vi "Angle_RT_test.vi"() -> ()   [LabVIEW 2021]
uses:
  <vilib>/DAQmx/read.llb/DAQmx Read (Digital 2D U32 NChan NSamp).vi
  <vilib>/Analysis/baseanly.llb/Mean (DBL).vi
  <vilib>/DAQmx/miscellaneous.llb/DAQmx Fill In Error Info.vi
  <vilib>/Analysis/NI_AALBase.lvlib
panel:
  out "Numeric":i32
  in  "stop":bool
  out "error out":errorcluster
  in  "Zero Angle":dbl[](array[numeric])=[-16.79, 2.64, -15.0, 3.7]
  out "Encoder Raw Outputs":dbl[][](array[numeric])
  out "Encoder Mean Outputs":dbl[](array[numeric])
  in  "Input Rate (Hz)":dbl
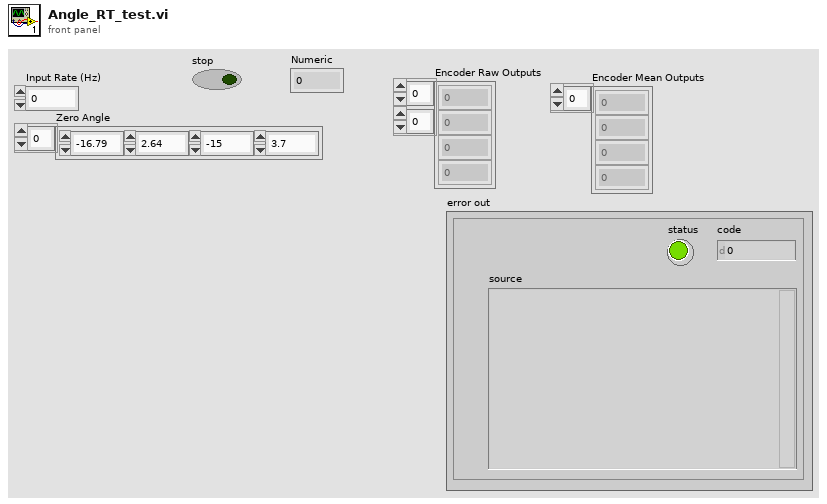
[diagram p1: front panel]
types:
  T1 = cluster{"Csn task out":refnum<k21>, "CLK task out":refnum<k21>, "D0 task out":refnum<k21>}
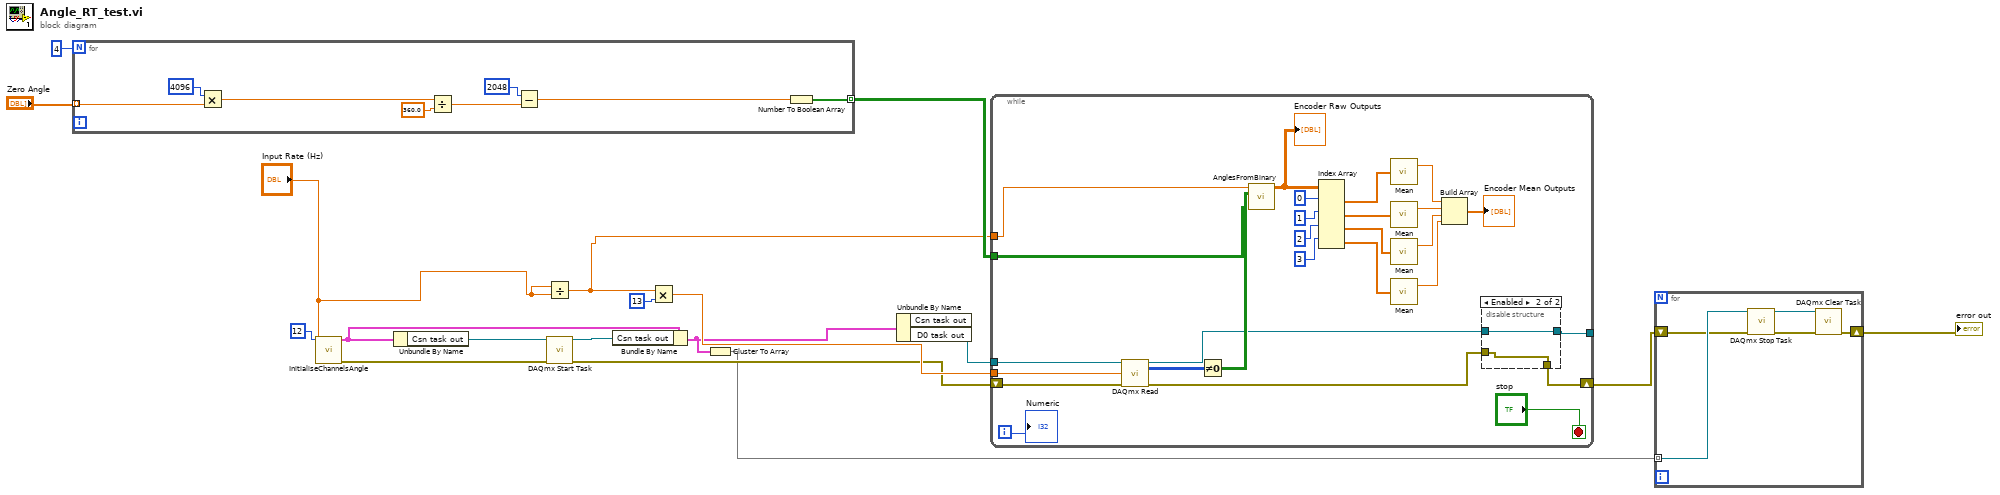
[diagram p0: block diagram]
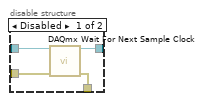
[diagram p2: hidden frame]
diagram:
  n1 = for {
    N: 4 -> [_]
    tunnel: [w22] -> w9 mode=indexing
    tunnel: "Zero Angle" -> [w25] mode=indexing
    n2 = Multiply(x=4096, y=w25) -> (x*y=w26:dbl)
    n3 = Divide(x=w26, y=360.0) -> (x/y=w20:dbl)
    n4 = Subtract(x=2048, y=w20) -> (x-y=w19:dbl)
    n5 = Number To Boolean Array(number=w19) -> (Boolean array=w22:bool[])
  }
  n6 = call "InitialiseChannelsAngle.vi"("Number of data bits"=12, "Fs"="Input Rate (Hz)") -> ("output cluster"=w13:T1, "error out"=w14:errorcluster)  [unwired: 12 in]
  n7 = Unbundle By Name(w13) -> ("Csn task out"=w18:refnum<k21>)
  n8 = Divide(x="Input Rate (Hz)", y="Input Rate (Hz)") -> (x/y=w8:dbl)
  n9 = call <vilib>:"DAQmx Start Task.vi"("task/channels in"=w18, "error in"=w14) -> ("task out"=w17:refnum<k21>, "error out"=w6:errorcluster)  [unwired: 12 in]
  n10 = Bundle By Name(cluster=w13, "Csn task out"=w17) -> (w2:T1)
  n11 = Multiply(x=w8, y=13) -> (x*y=w7:dbl)
  n12 = Cluster To Array(cluster=w2) -> (array=w4:refnum<k21>[])
  n13 = Unbundle By Name(w2) -> ("D0 task out"=w1:refnum<k21>)  [unwired: 1 out]
  n14 = while {
    tunnel: w9 -> [w37]
    tunnel: w8 -> [w36]
    tunnel: w7 -> [w35]
    tunnel: w1 -> [w30]
    shift-right: [w31] -> w5
    shift-left: w6 -> [w34]
    tunnel: [w27] -> _
    i -> [w29]
    stop <- "stop" stop-if-true
    n15 = call-poly <vilib>:"DAQmx Read.vi"("task/channels in"=w30, "number of samples per channel"=w35, "error in"=w34) -> ("task out"=w28:refnum<k21>, "data"=w53:u32[][], "error out"=w32:errorcluster)  [unwired: 10 in]
    n16 = Not Equal To 0?(x=w53) -> (x != 0?=w38:bool[][])
    n17 = call "AnglesFromBinary.vi"("Binary Offset"=w37, "Array"=w38, "Buffer Length"=w36) -> ("Unwrapped Phase"=w52:dbl[][])  [unwired: 8 in]
    "Encoder Raw Outputs" <- w52
    n18 = Index Array(array=w52, index (row) #1=0 ("index (row)"), index (row) #2=1 ("index (row)"), index (row) #3=2 ("index (row)"), index (row) #4=3 ("index (row)")) -> (element #1=w47:dbl[], element #2=w46:dbl[], element #3=w45:dbl[], element #4=w44:dbl[])  [unwired: 4 in]
    n19 = call-poly <vilib>:"Mean.vi"("X"=w47) -> ("mean"=w40:dbl)  [unwired: 1 out]
    n20 = call-poly <vilib>:"Mean.vi"("X"=w46) -> ("mean"=w41:dbl)  [unwired: 1 out]
    n21 = call-poly <vilib>:"Mean.vi"("X"=w45) -> ("mean"=w42:dbl)  [unwired: 1 out]
    n22 = call-poly <vilib>:"Mean.vi"("X"=w44) -> ("mean"=w43:dbl)  [unwired: 1 out]
    n23 = Build Array(w40, w41, w42, w43) -> (→"Encoder Mean Outputs":dbl[])
    n24 = disable-structure shown="Enabled" {
      disable-tunnel: w32 -> [w57 w58]
      disable-tunnel: [w56 w58] -> w31
      disable-tunnel: [w55 w59] -> w27
      disable-tunnel: w28 -> [w54 w59]
      frame Disabled {
        n25 = call <vilib>:"DAQmx Wait For Next Sample Clock.vi"("task/channels in"=w54, "error in"=w57) -> ("task out"=w55:refnum<k21>, "error out"=w56:errorcluster)  [unwired: 11 in, 1 out]
      }
      frame Enabled {
      }
    }
    "Numeric" <- w29
  }
  n26 = for {
    tunnel: w4 -> [w64] mode=indexing
    shift-right: [w60] -> w3
    shift-left: w5 -> [w62]
    n27 = call <vilib>:"DAQmx Stop Task.vi"("task/channels in"=w64, "error in"=w62) -> ("task out"=w63:refnum<k21>, "error out"=w61:errorcluster)  [unwired: 12 in]
    n28 = call <vilib>:"DAQmx Clear Task.vi"("task in"=w63, "error in"=w61) -> ("error out"=w60:errorcluster)  [unwired: 13 in]
  }
  "error out" <- w3
